vi "Teleop (WHS-R0B-62L0BS1's conflicted copy 2013-02-18).vi"(10 "Match Info":T1={"Autonomous Elapsed Seconds"=0.0, "TeleOp Elapsed Seconds"=0.0, "Disabled Elapsed Seconds"=0.0, "Visited Autonomous"=FALSE, "Visited TeleOp"=FALSE, "Visited Disabled"=FALSE, "Autonomous Settings"={"Autonomous Style"=enum."Independent", "VI Refnum"=refnum}}, 11 "Call Context":T2) -> ()   [LabVIEW 2012]
doc: "This VI is called for each TeleOp packet received from the DS where the robot is not disabled. It is often used to read from the joysticks and update I/O or to update setpoints for timed control loops. It should complete and return within 20 milliseconds or it may miss DS packets."
uses:
  <vilib>/Rock Robotics/WPI/DriverStation/WPI_DriverStationDerivedRobotMode.ctl
  <vilib>/Rock Robotics/WPI/DriverStation/WPI_DriverStationMatch Info.ctl
  <vilib>/Rock Robotics/WPI/Solenoid/WPI_SolenoidValue.ctl
  Robot Global Data.vi
  <vilib>/Rock Robotics/WPI/Solenoid/WPI_SolenoidSetEnum.vi
  <vilib>/Rock Robotics/WPI/Joystick/WPI_JoystickGetSetRefNum.vi
  <vilib>/Rock Robotics/WPI/RobotDrive/WPI_RobotDriveGetSetRefNum.vi
panel:
  in  "t 2":dbl=0.4
  in  "t":dbl=0.4
  out "Numeric 1":dbl(slide) scale=0.0..100.0
  out "Boolean 2":bool
  out "Boolean 1":bool
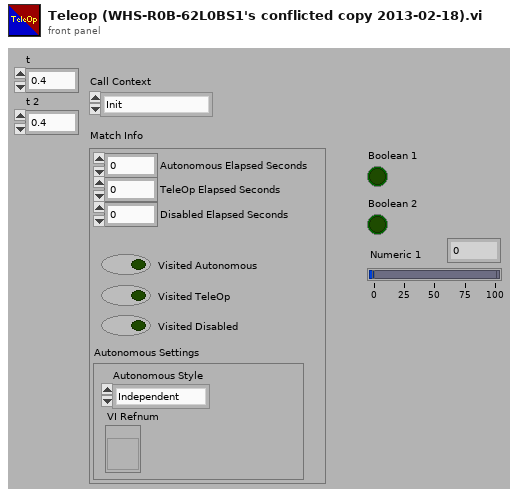
[diagram p1: front panel]
types:
  T1 = typedef "WPI_DriverStationMatch Info.ctl" = cluster{"Autonomous Elapsed Seconds":dbl, "TeleOp Elapsed Seconds":dbl, "Disabled Elapsed Seconds":dbl, "Visited Autonomous":bool, "Visited TeleOp":bool, "Visited Disabled":bool, "Autonomous Settings":cluster{"Autonomous Style":enum16{"Iterative", "Independent"}, "VI Refnum":refnum<vi>}}
  T2 = typedef "WPI_DriverStationDerivedRobotMode.ctl" = enum16{"Init", "Execute", "Stop"}
  T3 = typedef "WPI_SolenoidValue.ctl" = enum16{"Off", "On", "Forward", "Reverse"}
  T4 = typedef "WPI_JoystickDevRef.ctl" = cluster{"Device":T5}
  T5 = typedef "WPI_JoystickDeviceEnum.ctl" = enum16{"USB 1", "USB 2", "USB 3", "USB 4", "Kinect 1", "Kinect 2"}
  T6 = typedef "WPI_JoystickButtonState.ctl" = cluster{"Button 1":bool, "Button 2":bool, "Button 3":bool, "Button 4":bool, "Button 5":bool, "Button 6":bool, "Button 7":bool, "Button 8":bool, "Button 9":bool, "Button 10":bool, "Button 11":bool, "Button 12":bool}
  T7 = cluster{"axis 1 (x)":dbl, "axis 2 (y)":dbl, "axis 3 (throttle)":dbl, "axis 4":dbl, "axis 5":dbl, "axis 6":dbl}
  T8 = typedef "WPI_RobotDriveDevRef.ctl" = cluster{"DevStatus":errorcluster, "Motors[]":T9[], "Square Inputs":bool, "Max Output":dbl, "Isochronous":bool}
  T9 = typedef "WPI_MotorControlDeviceRef.ctl" = cluster{"DeviceStatus":errorcluster, "Type":enum16{"PWM", "CAN"}, "PWM":cluster{"Digital Module":T10, "PWM Channel":T11, "DeadBand":T12}, "CAN":cluster{"Device Number":u8, "Control Mode":T13, "Semaphore":T14, "Max Vout":dbl}, "Invert":bool, "TransformRef":T15, "InvTransformRef":T15}
  T10 = typedef "FPGA_TypedefDigitalModule.ctl" = enum16{"Digital Module 1", "Digital Module 2"}
  T11 = typedef "FPGA_DIOPWMChannel.ctl" = enum8{"PWM 1", "PWM 2", "PWM 3", "PWM 4", "PWM 5", "PWM 6", "PWM 7", "PWM 8", "PWM 9", "PWM 10", "Invalid"}
  T12 = typedef "WPI_PWMDeadband.ctl" = cluster{"Name":string, "maxPositivePwm":i32, "minPositivePwm":i32, "centerPwm":i32, "maxNegativePwm":i32, "minNegativePwm":i32, "angularRange":u16}
  T13 = typedef "WPI_CANJaguar_ControlMode.ctl" = enum8{"Percent VBus", "Current", "Speed", "Position", "Voltage"}
  T14 = typedef "Semaphore RefNum" = refnum<k1>
  T15 = typedef "WPI_PWMTransform_ConPane.ctl" = refnum<vi>
  T16 = typedef "WPI_SolenoidDevRef.ctl" = cluster{"DevStatus":errorcluster, "Solenoid Module":T17, "Forward Solenoid Channel":T18, "Reverse Solenoid Channel":T18}
  T17 = typedef "FPGA_TypedefSolenoidModule.ctl" = enum16{"Solenoid Module 1", "Solenoid Module 2"}
  T18 = typedef "WPI_SolenoidChannel.ctl" = enum8{"Solenoid 1", "Solenoid 2", "Solenoid 3", "Solenoid 4", "Solenoid 5", "Solenoid 6", "Solenoid 7", "Solenoid 8", "Invalid"}
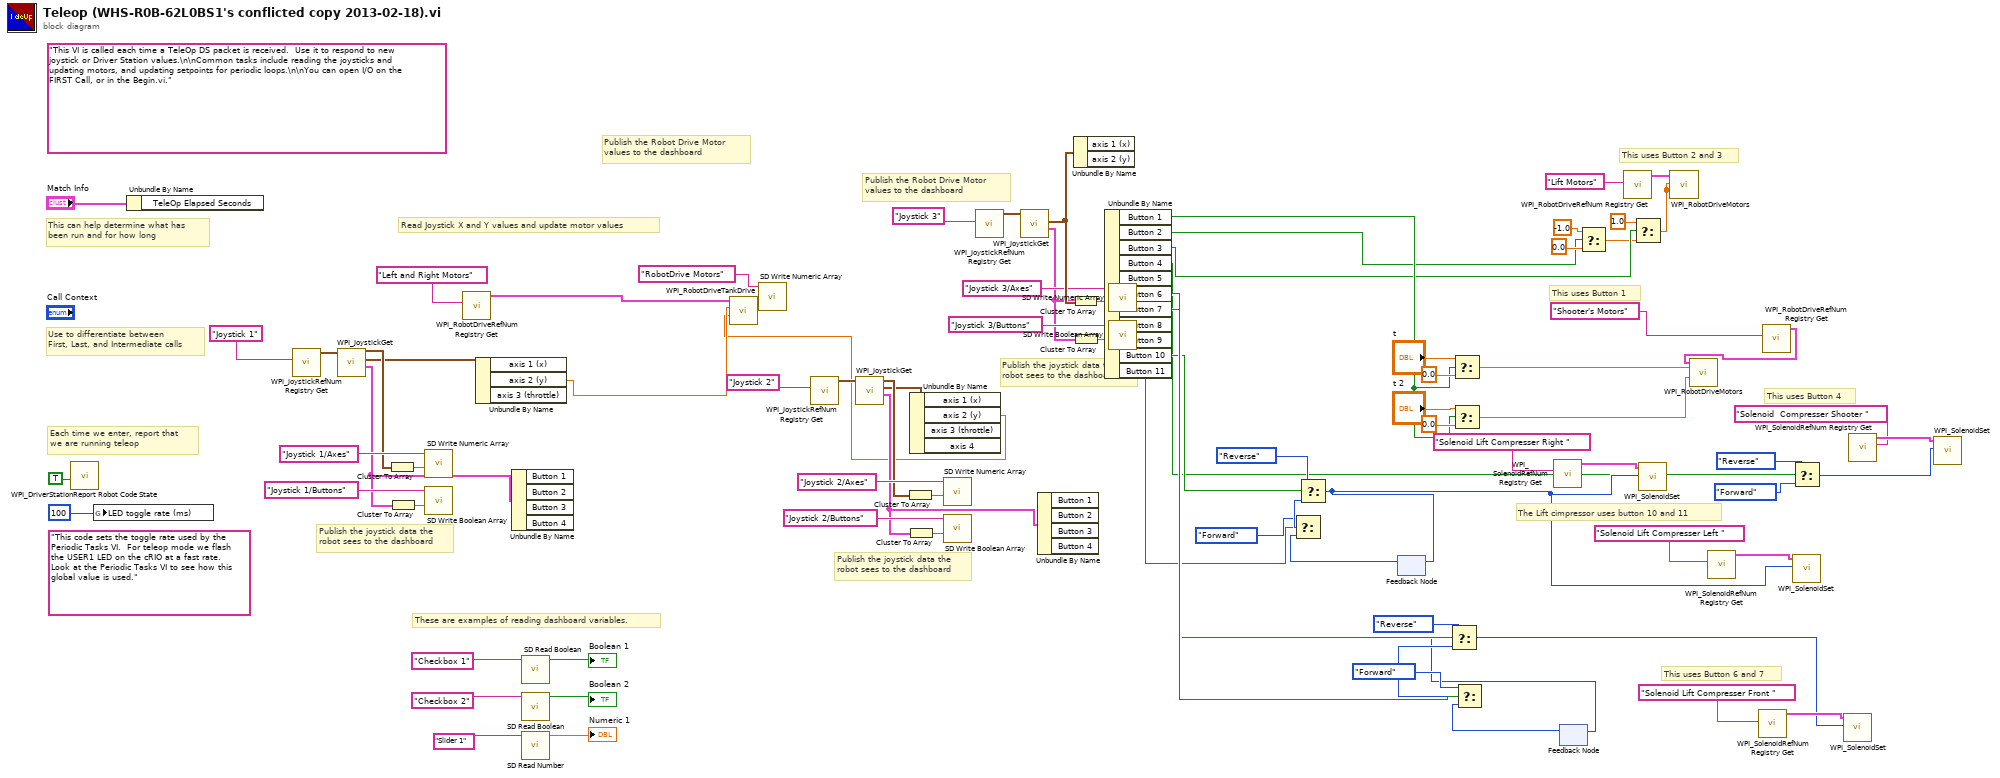
[diagram p0: block diagram]
diagram:
  (unwired) "This code sets the toggle rate used by the Periodic Tasks VI.  For teleop mode we flash the USER1 LED on the cRIO at a fast rate.  Look at the Periodic Tasks VI to see how this global value is used."
  (unwired) "This VI is called each time a TeleOp DS packet is received.  Use it to respond to new joystick or Driver Station values.\n\nCommon tasks include reading the joysticks and updating motors, and updating setpoints for periodic loops.\n\nYou can open I/O on the FIRST Call, or in the Begin.vi."
  # "This uses Button 2 and 3"
  # "The Lift cimpressor uses button 10 and 11"
  # "This uses Button 1"
  # "This uses Button 6 and 7"
  # "This uses Button 4"
  # "Publish the joystick data the\nrobot sees to the dashboard"
  # "Publish the Robot Drive Motor\nvalues to the dashboard"
  # "Publish the joystick data the\nrobot sees to the dashboard"
  # "These are examples of reading dashboard variables."
  # "Publish the Robot Drive Motor\nvalues to the dashboard"
  # "Publish the joystick data the\nrobot sees to the dashboard"
  # "Each time we enter, report that\nwe are running teleop"
  # "Use to differentiate between\nFirst, Last, and Intermediate calls"
  # "This can help determine what has\nbeen run and for how long"
  # "Read Joystick X and Y values and update motor values"
  n1 = call <vilib>:"WPI_DriverStationReport Robot Code State.vi"("TeleOp"=TRUE ("Autonomous")) -> ()  [unwired: 10 in, 1 out]
  n2 = global write "Robot Global Data.vi" "LED toggle rate (ms)"(u32 100 ("LED ms toggle rate")) -> ()
  n3 = Unbundle By Name("Match Info") -> ()  [unwired: 1 out]
  n4 = call <vilib>:"WPI_JoystickRefNum Registry Get.vi"("refnum name"="Joystick 1") -> ("JoystickDevRef"=w81:T4)  [unwired: 1 in, 9 out]
  n5 = call <vilib>:"WPI_JoystickGet.vi"("JoystickDevRef"=w81) -> ("Buttons"=w32:T6, "Axes"=w29:T7, "JoystickDevRef"=w34:T4)  [unwired: 1 in, 3 out]
  n6 = Cluster To Array(cluster=w34) -> (array=w76:T5[])
  n7 = Cluster To Array(cluster=w32) -> (array=w78:bool[])
  n8 = call <vilib>:"SD Write Numeric Array.vi"("Numeric Array"=w76, "Name"="Joystick 1/Axes") -> ()  [unwired: 8 in, 2 out]
  n9 = call <vilib>:"SD Write Boolean Array.vi"("Boolean Array"=w78, "Name"="Joystick 1/Buttons") -> ()  [unwired: 8 in, 2 out]
  n10 = call <vilib>:"WPI_RobotDriveRefNum Registry Get.vi"("refnum name"="Left and Right Motors") -> ("RobotDriveDevRef"=w83:T8)  [unwired: 1 in, 9 out]
  n11 = Unbundle By Name(w29) -> ("axis 2 (y)"=w28:dbl)  [unwired: 2 out]
  n12 = Unbundle By Name(w32) -> ()  [unwired: 4 out]
  n13 = call <vilib>:"SD Read Boolean.vi"("Name"="Checkbox 1" ("refnum name")) -> ("Boolean"=→"Boolean 1":bool)  [unwired: 8 in, 2 out]
  n14 = call <vilib>:"SD Read Boolean.vi"("Name"="Checkbox 2" ("refnum name")) -> ("Boolean"=→"Boolean 2":bool)  [unwired: 8 in, 2 out]
  n15 = call <vilib>:"SD Read Number.vi"("Name"="Slider 1" ("refnum name")) -> ("Numeric"=→"Numeric 1":dbl)  [unwired: 8 in, 2 out]
  n16 = call <vilib>:"WPI_JoystickRefNum Registry Get.vi"("refnum name"="Joystick 2") -> ("JoystickDevRef"=w63:T4)  [unwired: 1 in, 9 out]
  n17 = call <vilib>:"WPI_JoystickGet.vi"("JoystickDevRef"=w63) -> ("Buttons"=w31:T6, "Axes"=w30:T7, "JoystickDevRef"=w33:T4)  [unwired: 1 in, 3 out]
  n18 = Cluster To Array(cluster=w33) -> (array=w35:T5[])
  n19 = Cluster To Array(cluster=w31) -> (array=w64:bool[])
  n20 = Unbundle By Name(w30) -> ("axis 2 (y)"=w27:dbl)  [unwired: 3 out]
  n21 = call <vilib>:"WPI_RobotDriveTankDrive.vi"("Right axis value"=w27, "Left axis value"=w28, "RobotDriveDevRef"=w83) -> ("Motor Values"=w73:dbl[])  [unwired: 6 in, 2 out]
  n22 = call <vilib>:"SD Write Numeric Array.vi"("Numeric Array"=w73, "Name"="RobotDrive Motors") -> ()  [unwired: 8 in, 2 out]
  n23 = call <vilib>:"SD Write Numeric Array.vi"("Numeric Array"=w35, "Name"="Joystick 2/Axes") -> ()  [unwired: 8 in, 2 out]
  n24 = call <vilib>:"SD Write Boolean Array.vi"("Boolean Array"=w64, "Name"="Joystick 2/Buttons") -> ()  [unwired: 8 in, 2 out]
  n25 = call <vilib>:"WPI_JoystickRefNum Registry Get.vi"("refnum name"="Joystick 3") -> ("JoystickDevRef"=w60:T4)  [unwired: 1 in, 9 out]
  n26 = call <vilib>:"WPI_JoystickGet.vi"("JoystickDevRef"=w60) -> ("Buttons"=w54:T6, "Axes"=w57:T7)  [unwired: 1 in, 4 out]
  n27 = Unbundle By Name(w31) -> ()  [unwired: 4 out]
  n28 = Cluster To Array(cluster=w57) -> (array=w56:dbl[])
  n29 = Cluster To Array(cluster=w54) -> (array=w59:bool[])
  n30 = Unbundle By Name(w57) -> ()  [unwired: 2 out]
  n31 = Unbundle By Name(w54) -> ("Button 1"=w49:bool, "Button 2"=w40:bool, "Button 3"=w41:bool, "Button 4"=w1:bool, "Button 6"=w19:bool, "Button 7"=w18:bool, "Button 10"=w8:bool, "Button 11"=w7:bool)  [unwired: 3 out]
  n32 = call <vilib>:"SD Write Numeric Array.vi"("Numeric Array"=w56, "Name"="Joystick 3/Axes") -> ()  [unwired: 8 in, 2 out]
  n33 = call <vilib>:"SD Write Boolean Array.vi"("Boolean Array"=w59, "Name"="Joystick 3/Buttons") -> ()  [unwired: 8 in, 2 out]
  n34 = feedback #1() -> (w13:T3)  [unwired: 1 in]
  n35 = Select(t=WPI_SolenoidValue."Forward" ("Value"), s=w7, f=w13) -> (s? t:f=w12:T3)
  n36 = Select(t=WPI_SolenoidValue."Reverse" ("Value"), s=w8, f=w12) -> (s? t:f=w9:T3)
  n37 = feedback-in #1(w9) -> ()
  n38 = Select(t="t", s=w49, f=0.0) -> (s? t:f=w47:dbl)
  n39 = Select(t="t 2", s=w49, f=0.0) -> (s? t:f=w48:dbl)
  n40 = call <vilib>:"WPI_SolenoidRefNum Registry Get.vi"("refnum name"="Solenoid Lift Compresser Right ") -> ("SolenoidDevRef"=w25:T16)  [unwired: 9 in, 1 out]
  n41 = feedback #2() -> (w14:T3)  [unwired: 1 in]
  n42 = Select(t=WPI_SolenoidValue."Forward" ("Value"), s=w19, f=w14) -> (s? t:f=w16:T3)
  n43 = Select(t=WPI_SolenoidValue."Reverse" ("Value"), s=w18, f=w16) -> (s? t:f=w15:T3)
  n44 = feedback-in #2(w15) -> ()
  n45 = Select(t=-1.0, s=w40, f=0.0) -> (s? t:f=w39:dbl)
  n46 = call <vilib>:"WPI_RobotDriveRefNum Registry Get.vi"("refnum name"="Lift Motors") -> ("RobotDriveDevRef"=w37:T8)  [unwired: 9 in, 1 out]
  n47 = Select(t=1.0, s=w41, f=w39) -> (s? t:f=w36:dbl)
  n48 = call-poly <vilib>:"WPI_SolenoidSet.vi"("Value"=w9, "SolenoidDevRef"=w25) -> ()  [unwired: 8 in, 2 out]
  n49 = call <vilib>:"WPI_RobotDriveMotors.vi"("RightSpeed"=w36, "LeftSpeed"=w36, "RobotDriveDevRef"=w37) -> ()  [unwired: 1 in, 8 out]
  n50 = call <vilib>:"WPI_SolenoidRefNum Registry Get.vi"("refnum name"="Solenoid Lift Compresser Left ") -> ("SolenoidDevRef"=w24:T16)  [unwired: 9 in, 1 out]
  n51 = call <vilib>:"WPI_SolenoidRefNum Registry Get.vi"("refnum name"="Solenoid Lift Compresser Front ") -> ("SolenoidDevRef"=w20:T16)  [unwired: 9 in, 1 out]
  n52 = call <vilib>:"WPI_RobotDriveRefNum Registry Get.vi"("refnum name"="Shooter's Motors") -> ("RobotDriveDevRef"=w45:T8)  [unwired: 9 in, 1 out]
  n53 = call <vilib>:"WPI_RobotDriveMotors.vi"("RightSpeed"=w48, "LeftSpeed"=w47, "RobotDriveDevRef"=w45) -> ()  [unwired: 1 in, 8 out]
  n54 = call-poly <vilib>:"WPI_SolenoidSet.vi"("Value"=w9, "SolenoidDevRef"=w24) -> ()  [unwired: 8 in, 2 out]
  n55 = Select(t=WPI_SolenoidValue."Reverse" ("Value"), s=w1, f=WPI_SolenoidValue."Forward" ("Value")) -> (s? t:f=w2:T3)
  n56 = call-poly <vilib>:"WPI_SolenoidSet.vi"("Value"=w15, "SolenoidDevRef"=w20) -> ()  [unwired: 8 in, 2 out]
  n57 = call <vilib>:"WPI_SolenoidRefNum Registry Get.vi"("refnum name"="Solenoid  Compresser Shooter ") -> ("SolenoidDevRef"=w6:T16)  [unwired: 9 in, 1 out]
  n58 = call-poly <vilib>:"WPI_SolenoidSet.vi"("Value"=w2, "SolenoidDevRef"=w6) -> ()  [unwired: 8 in, 2 out]
